vi "LinearPidTuningPanel.vi"() -> ()   [LabVIEW 2014]
uses:
  <vilib>/silver_ctls/ArrayMatrixCluster/Real Matrix NI_Silver.ctl
panel:
  in  "Update Ki":bool=TRUE
  in  "Update Kd":bool=TRUE
  in  "Update Kp":bool=TRUE
  in  "Matrix Type":u16(ring) items=["Diagonal", "Normal"]
  out "Output":string
  in  "Ki":T1=[[1.0, 0.0, 0.0, 0.0, 0.0, 0.0], [0.0, 1.0, 0.0, 0.0, 0.0, 0.0], [0.0, 0.0, 1.0, 0.0, 0.0, 0.0], [0.0, 0.0, 0.0, 1.0, 0.0, 0.0], [0.0, 0.0, 0.0, 0.0, 1.0, 0.0], [0.0, 0.0, 0.0, 0.0, 0.0, 1.0]]
  in  "Kd":T1=[[1.0, 0.0, 0.0, 0.0, 0.0, 0.0], [0.0, 1.0, 0.0, 0.0, 0.0, 0.0], [0.0, 0.0, 1.0, 0.0, 0.0, 0.0], [0.0, 0.0, 0.0, 1.0, 0.0, 0.0], [0.0, 0.0, 0.0, 0.0, 1.0, 0.0], [0.0, 0.0, 0.0, 0.0, 0.0, 1.0]]
  in  "Kp":T1=[[1.0, 0.0, 0.0, 0.0, 0.0, 0.0], [0.0, 1.0, 0.0, 0.0, 0.0, 0.0], [0.0, 0.0, 1.0, 0.0, 0.0, 0.0], [0.0, 0.0, 0.0, 1.0, 0.0, 0.0], [0.0, 0.0, 0.0, 0.0, 1.0, 0.0], [0.0, 0.0, 0.0, 0.0, 0.0, 1.0]]
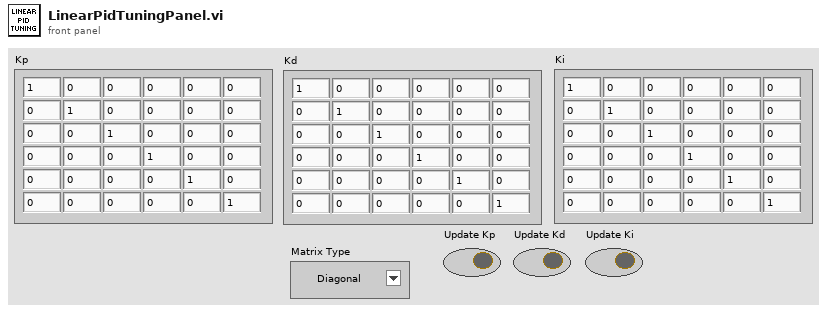
[diagram p1: front panel]
types:
  T1 = typedef "Real Matrix NI_Silver.ctl" = dbl[][]
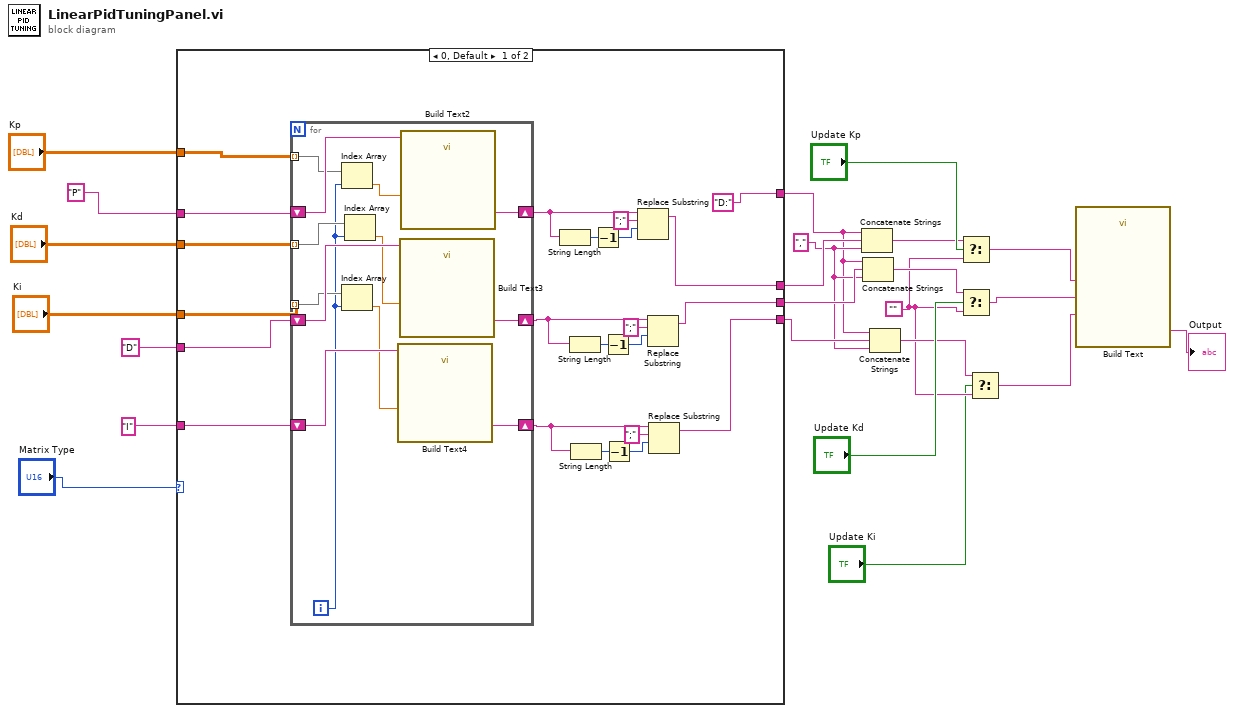
[diagram p0: block diagram]
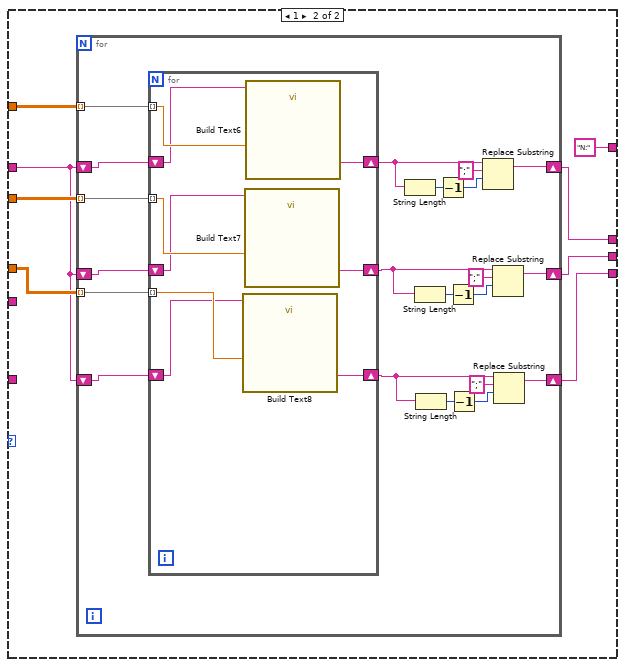
[diagram p2: hidden frame]
diagram:
  w3 = ""
  w12 = ","
  n1 = case shown="0, Default" "Matrix Type" {
    tunnel: "Kp" -> [w33 w66]
    tunnel: "Kd" -> [w32 w65]
    tunnel: "Ki" -> [w31 w64]
    tunnel: "P" -> [w27 w63]
    tunnel: [w30 w62] -> w15
    tunnel: [w29 w61] -> w14
    tunnel: [w28 w60] -> w13
    tunnel: "D" -> [w26 _]
    tunnel: "I" -> [w25 _]
    tunnel: ["D:" "N:"] -> w11
    frame 0, Default {
      n2 = for {
        tunnel: w33 -> [w52] mode=indexing
        shift-right: [w58] -> w34
        shift-left: w25 -> [w57]
        shift-right: [w56] -> w35
        shift-left: w26 -> [w55]
        shift-right: [w54] -> w45
        shift-left: w27 -> [w53]
        tunnel: w32 -> [w50] mode=indexing
        tunnel: w31 -> [w48] mode=indexing
        i -> [w46]
        n3 = Index Array(array=w52, index=w46) -> (element=w51:dbl)
        n4 = Index Array(array=w48, index=w46) -> (element=w47:dbl)
        n5 = Index Array(array=w50, index=w46) -> (element=w49:dbl)
        n6 = call "Build Text4"("Beginning Text"=w57, "Elem"=w47) -> ("Result"=w58:string)  [unwired: 12 in, 1 out]
        n7 = call "Build Text3"("Beginning Text"=w55, "Elem"=w49) -> ("Result"=w56:string)  [unwired: 12 in, 1 out]
        n8 = call "Build Text2"("Beginning Text"=w53, "Elem"=w51) -> ("Result"=w54:string)  [unwired: 12 in, 1 out]
      }
      n9 = String Length(string=w45) -> (length=w43:i32)
      n10 = String Length(string=w35) -> (length=w40:i32)
      n11 = String Length(string=w34) -> (length=w37:i32)
      n12 = Decrement(x=w43) -> (x-1=w42:i32)
      n13 = Decrement(x=w40) -> (x-1=w39:i32)
      n14 = Decrement(x=w37) -> (x-1=w36:i32)
      n15 = Replace Substring(3:w42, 4:";" ("substring (\"\")"), 5:w45) -> (1:w30:string)  [unwired: 1 in, 1 out]
      n16 = Replace Substring(3:w39, 4:";" ("substring (\"\")"), 5:w35) -> (1:w29:string)  [unwired: 1 in, 1 out]
      n17 = Replace Substring(3:w36, 4:";" ("substring (\"\")"), 5:w34) -> (1:w28:string)  [unwired: 1 in, 1 out]
    }
    frame 1 {
      n18 = for {
        tunnel: w66 -> [w87] mode=indexing
        tunnel: w65 -> [w86] mode=indexing
        tunnel: w64 -> [w85] mode=indexing
        shift-right: [w80] -> w62
        shift-left: w63 -> [w79]
        shift-right: [w71] -> w61
        shift-left: w63 -> [w70]
        shift-right: [w69] -> w60
        shift-left: w63 -> [w68]
        n19 = for {
          tunnel: w87 -> [w96] mode=indexing
          tunnel: w86 -> [w95] mode=indexing
          tunnel: w85 -> [w94] mode=indexing
          shift-right: [w93] -> w67
          shift-left: w68 -> [w92]
          shift-right: [w91] -> w72
          shift-left: w70 -> [w90]
          shift-right: [w89] -> w84
          shift-left: w79 -> [w88]
          n20 = call "Build Text8"("Beginning Text"=w92, "Elem"=w94) -> ("Result"=w93:string)  [unwired: 12 in, 1 out]
          n21 = call "Build Text7"("Beginning Text"=w90, "Elem"=w95) -> ("Result"=w91:string)  [unwired: 12 in, 1 out]
          n22 = call "Build Text6"("Beginning Text"=w88, "Elem"=w96) -> ("Result"=w89:string)  [unwired: 12 in, 1 out]
        }
        n23 = String Length(string=w84) -> (length=w82:i32)
        n24 = String Length(string=w72) -> (length=w77:i32)
        n25 = String Length(string=w67) -> (length=w74:i32)
        n26 = Decrement(x=w82) -> (x-1=w81:i32)
        n27 = Decrement(x=w77) -> (x-1=w76:i32)
        n28 = Decrement(x=w74) -> (x-1=w73:i32)
        n29 = Replace Substring(3:w81, 4:";" ("substring (\"\")"), 5:w84) -> (1:w80:string)  [unwired: 1 in, 1 out]
        n30 = Replace Substring(3:w76, 4:";" ("substring (\"\")"), 5:w72) -> (1:w71:string)  [unwired: 1 in, 1 out]
        n31 = Replace Substring(3:w73, 4:";" ("substring (\"\")"), 5:w67) -> (1:w69:string)  [unwired: 1 in, 1 out]
      }
    }
  }
  n32 = Concatenate Strings(w11, w15, w12) -> (w9:string)
  n33 = Concatenate Strings(w11, w14, w12) -> (w7:string)
  n34 = Concatenate Strings(w11, w13, w12) -> (w4:string)
  n35 = Select(t=w9, s="Update Kp", f=w3) -> (s? t:f=w8:string)
  n36 = Select(t=w7, s="Update Kd", f=w3) -> (s? t:f=w5:string)
  n37 = Select(t=w4, s="Update Ki", f=w3) -> (s? t:f=w1:string)
  n38 = call "Build Text"("Kp"=w8, "Kd"=w5, "Ki"=w1) -> ("Result"=→"Output":string)  [unwired: 11 in, 1 out]
